vi "ScanQueueRecalc Value Change.vi"(9 "Queue Size":u16=2, 10 "Scans Per Write":u16=20, 11 "References":T1) -> (0 "error out":errorcluster, 2 "Approximate Memory Usage":dbl)   [LabVIEW 2015, in "TDMS datalogger editor node.lvclass"]
uses:
  TDMS datalogger editor node.lvclass
  <vilib>/NI/DCAF/Tag Editor Core/Table API/Table Manager/object ref.ctl
  <vilib>/NI/DCAF/Tag Editor Core/Configuration Editor/Classes/Engine Parent/Engine Parent Editor Node.lvclass
  <vilib>/NI/DCAF/Tag Editor Core/Configuration Editor/Classes/Module editor node/module editor node.lvclass
  TDMS datalogger editor node.lvclass/TDMS datalogger editor node.ctl
  module/configuration/TDMS datalogger configuration.lvclass/TDMS datalogger configuration.ctl
  <vilib>/NI/Tag Bus/tag/tag descriptor.lvclass/tag descriptor.ctl
  module/configuration/Write scans per write.vi
  module/configuration/Write queue size.vi
  module/configuration/TDMS datalogger configuration.lvclass
  <vilib>/NI/Tag Bus/tag/tag descriptor.lvclass
  <vilib>/NI/DCAF/Tag Editor Core/Table API/Table Manager/Table Manager.lvclass
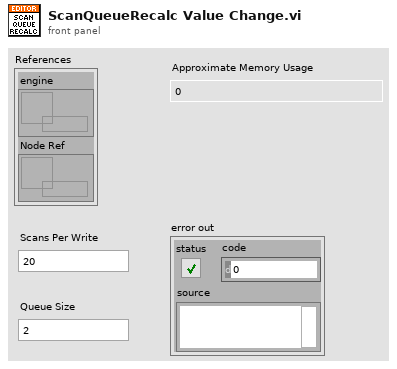
[diagram p1: front panel]
types:
  T1 = typedef "Table Manager.lvlib/Table Manager.lvclass/object ref.ctl" = cluster{"engine":refnum<data-value>, "Node Ref":refnum<data-value>}
  T2 = typedef "tag bus.lvlib/tag descriptor.lvclass/Data Type.ctl" = enum16{"Double", "Single", "I64", "I32", "I16", "I8", "U64", "U32", "U16", "U8", "Boolean", "String", "Array of Double", "Array of Single", "Array of I64", "Array of I32", "Array of I16", "Array of I8", "Array of U64", "Array of U32", "Array of U16", "Array of U8", "Array of Boolean", "Array of String"}
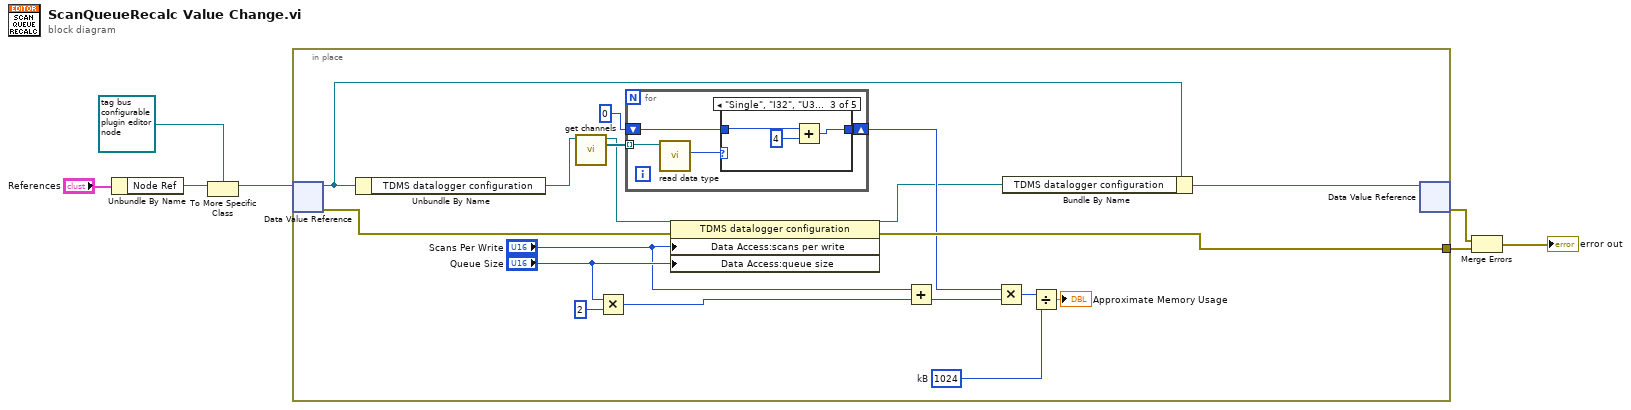
[diagram p0: block diagram]
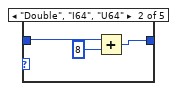
[diagram p3: hidden frame]
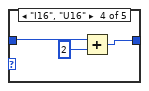
[diagram p4: hidden frame]
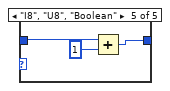
[diagram p5: hidden frame]
diagram:
  n1 = Unbundle By Name("References") -> ("Node Ref"=w6:refnum<data-value>)
  n2 = To More Specific Class(target class=refnum<data-value> refnum ("data value reference"), reference=w6) -> (specific class reference=w4:refnum<data-value>)  [unwired: 1 in, 1 out]
  n3 = in-place {
    in-place-border: [w25] -> w3
    w22 = u32 1024  # kB
    n4 = in-place-dvr #1(w4) -> (w15:refnum<class "TDMS datalogger editor node.lvclass">, w16:errorcluster)
    n5 = Unbundle By Name(w15) -> ("TDMS datalogger configuration"=w13:refnum<class "TDMS datalogger configuration.lvclass">)
    n6 = call-dynamic "get channels.vi"("module configuration in"=w13) -> ("channels"=w19:refnum<class "TBM channel.lvclass">[], "module configuration out"=w17:refnum<class "TDMS datalogger configuration.lvclass">)  [unwired: 9 in]
    n7 = Multiply(x="Queue Size", y=2 ("x")) -> (x*y=w9:i32)
    n8 = for {
      shift-right: [w28] -> w20
      shift-left: u32 0 -> [w29]
      tunnel: w19 -> [w26] mode=indexing
      n9 = call <vilib>:"read data type.vi"("system tag in"=w26) -> ("data type"=w27:T2)  [unwired: 8 in, 2 out]
      n10 = case shown="\"Single\", \"I32\", \"U32\"" w27 {
        tunnel: w29 -> [w30 w33 w36 w39 w42]
        tunnel: [w30 w32 w35 w38 w41] -> w28
        frame Default {
        }
        frame "Double", "I64", "U64" {
          n11 = Add(x=w33, y=u32 8) -> (x+y=w32:u32)
        }
        frame "Single", "I32", "U32" {
          n12 = Add(x=w36, y=u32 4) -> (x+y=w35:u32)
        }
        frame "I16", "U16" {
          n13 = Add(x=w39, y=u32 2) -> (x+y=w38:u32)
        }
        frame "I8", "U8", "Boolean" {
          n14 = Add(x=w42, y=u32 1) -> (x+y=w41:u32)
        }
      }
    }
    n15 = property class="TDMS datalogger configuration"(reference=w17, error in=w16, "Data Access:scans per write"="Scans Per Write", "Data Access:queue size"="Queue Size") -> (reference out=w12:refnum<class "TDMS datalogger configuration.lvclass">, error out=w25:errorcluster)
    n16 = Add(x="Scans Per Write", y=w9) -> (x+y=w10:i32)
    n17 = Multiply(x=w20, y=w10) -> (x*y=w11:u32)
    n18 = Bundle By Name(cluster=w15, "TDMS datalogger configuration"=w12) -> (w14:refnum<class "TDMS datalogger editor node.lvclass">)
    n19 = Divide(x=w11, y=w22) -> (x/y=→"Approximate Memory Usage":dbl)
    n20 = in-place-dvr #1(w14) -> (w1:errorcluster)  [unwired: 1 out]
  }
  n21 = Merge Errors(w1, w3) -> (→"error out":errorcluster)
